vi "Reading Temperature Data.vi"() -> ()   [LabVIEW 2017]
panel:
  in  "Stop Button":bool
  out "Temperature Data":dbl format="%.1g"
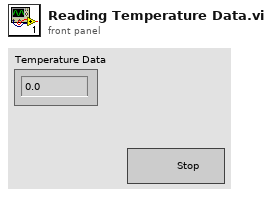
[diagram p1: front panel]
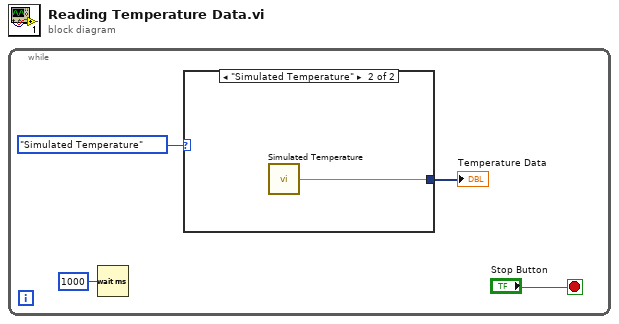
[diagram p0: block diagram]
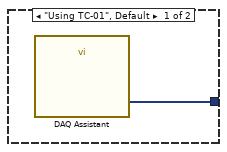
[diagram p2: hidden frame]
diagram:
  n1 = while {
    stop <- "Stop Button" stop-if-true
    n2 = Wait (ms)(milliseconds to wait=u32 1000) -> ()  [unwired: 1 out]
    n3 = case shown="\"Simulated Temperature\"" enum16{"Using TC-01", "Simulated Temperature"}."Simulated Temperature" ("Enum") {
      tunnel: [w5 w6] -> w4
      frame "Using TC-01", Default {
        n4 = call "DAQ Assistant"() -> ("data"=w5:dynamicdata)  [unwired: 17 in, 2 out]
      }
      frame "Simulated Temperature" {
        n5 = call "Simulated Temperature.vi"() -> ("Temperature Value"=w6:dbl)  [unwired: 2 in]
      }
    }
    "Temperature Data" <- w4
  }
